vi "Configure Edge Trigger.vi"(0 "device session in":refnum<class "Device Session.lvclass">, 1 "trigger source":u8, 5 "trigger slope":T1, 7 "trigger level (V)":dbl, 9 "hysteresis (%fs)":dbl=0.25, 11 "error in":errorcluster, 12 "instance":enum16{"A", "B"}(ring)) -> (4 "device session out":refnum<class "Device Session.lvclass">, 15 "error out":errorcluster)   [LabVIEW 2021, in "Device Session.lvclass"]
doc: "Configures the edge trigger for the selected channel. You can specify the trigger level, hysteresis, and trigger slope.\n\n<B>Input Parameters</B>\n\n<B>device session in</B> is a reference to the Device Session object, which contains a session to each instrument design library used in this sample project. This parameter is obtained from the 'Open Session' VI.\n\n<B>trigger source</B> specifies the channel to monitor for trigger conditions.\n\n<B>trigger slope</B> specifies whether the oscilloscope should trigger on a rising edge or a falling edge.\n\n<B>trigger level (V)</B> specifies the voltage threshold for the trigger.\n\n<B>hysteresis (%fs)</B> specifies in volts the size of the hysteresis window on either side of the specified 'level'. The oscilloscope triggers when the 'trigger source' signal passes through the 'hysteresis level' you specify with this parameter, has the specified 'trigger slope', and passes through the specified 'level'.\n\n<B>instance</B> specifies either instance A or B of the trigger to use.\n\n<B>error in</B> describes error conditions that occur before this node runs. This input provides standard 'error in' functionality.\n\n<B>Output Parameters</B>\n\n<B>device session out</B> passes a reference to the session to the next VI.\n\n<B>error out</B> contains error information. This output provides standard 'error out' functionality."
uses:
  Device Session.lvclass
  <instrlib>/_niInstr/Data Trigger/v1/Shared/Public/Edge Configuration Trigger Slope.ctl
  Device Session.lvclass/Device Session.ctl
  <instrlib>/_niInstr/Data Trigger/v1/Shared/Public/Edge Configuration FXP(+-,18,1).ctl
  FPGA Refnum.ctl
  <vilib>/rvi/interface/nirviReadWriteControl/nirviReadWriteControl.xnode
  <vilib>/rvi/interface/Simulation/niFpgaSimulationCallBeginRW.vi
  <vilib>/rvi/errors/niLvFpgaAdjustHostInterfaceError.vi
  <instrlib>/_niInstr/Data Trigger/v1/Shared/niInstr Data Trigger v1 Shared.lvlib
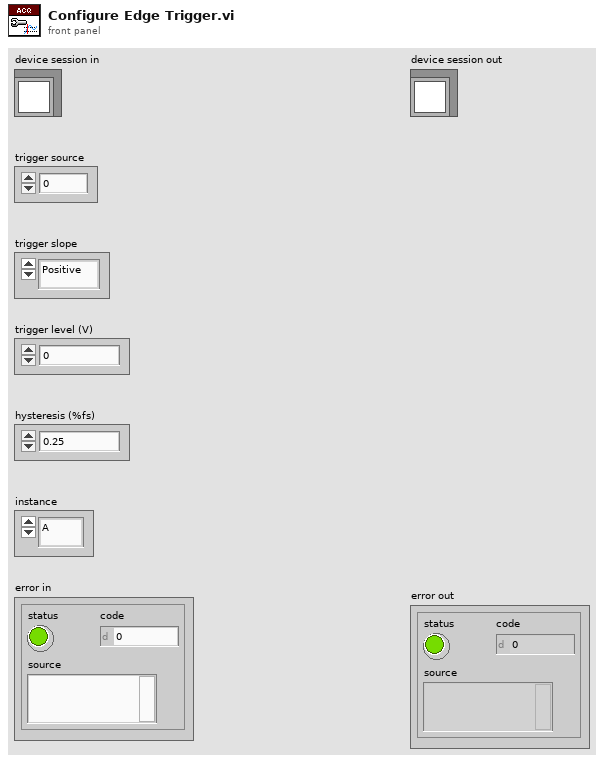
[diagram p1: front panel]
types:
  T1 = typedef "niInstr Data Trigger v1 Shared.lvlib/Edge Configuration Trigger Slope.ctl" = enum8{"Positive", "Negative"}
  T2 = typedef "niInstr Data Trigger v1 Shared.lvlib/Edge Configuration FXP(+-,18,1).ctl" = cluster{"highLevel":fxp<+/-,18,1>, "lowLevel":fxp<+/-,18,1>, "trigger slope":T1}
  T3 = typedef "Device Session.lvclass/Device Session Object.ctl" = cluster{"fpga reference":T4, "reg bus":refnum<class "niInstr FIFO Register Bus v1 Host.lvclass">, "subsystem map":refnum<class "niInstr Subsystem Map v1 Host.lvclass">, "cal data":refnum<class "niHSAI Cal Data v1 Host.lvclass">, "config":refnum<class "niHSAI Group A Config v1 Host.lvclass">, "acquisition":refnum<class "niInstr Multirecord Acquisition v1 Host.lvclass">, "number of selected acq channels":u8, "selected acq channels":bool[], "number of channels":u32, "configured channels":bool[], "acq configuration":cluster{"number of samples":u64, "number of records":u64, "pretrigger samples":u64}, "actual channel configuration":T5[], "sample clock rate (Hz)":dbl, "scaling coefficients":T9[]}
  T4 = typedef "Device Session.lvclass/FPGA Refnum.ctl" = refnum<k20>
  T5 = typedef "niHSAI Types v1 Host.lvlib/Channel Configuration.ctl" = cluster{"channel":u32, "coupling":T6, "impedance":T7, "bandwidth":T8, "vertical range":dbl, "vertical offset":dbl}
  T6 = typedef "niHSAI Types v1 Host.lvlib/Coupling.ctl" = enum8{"Default", "DC", "AC"}
  T7 = typedef "niHSAI Types v1 Host.lvlib/Impedance.ctl" = enum8{"Default", "1 mega ohm", "50 ohm"}
  T8 = typedef "niHSAI Types v1 Host.lvlib/Bandwidth.ctl" = enum8{"Default", "Full Bandwidth", "Anti-alias Filter", "150 MHz"}
  T9 = typedef "niInstr Multirecord Acquisition v1 Host.lvclass/Scaling Coefficient.ctl" = cluster{"gain":dbl, "offset":dbl}
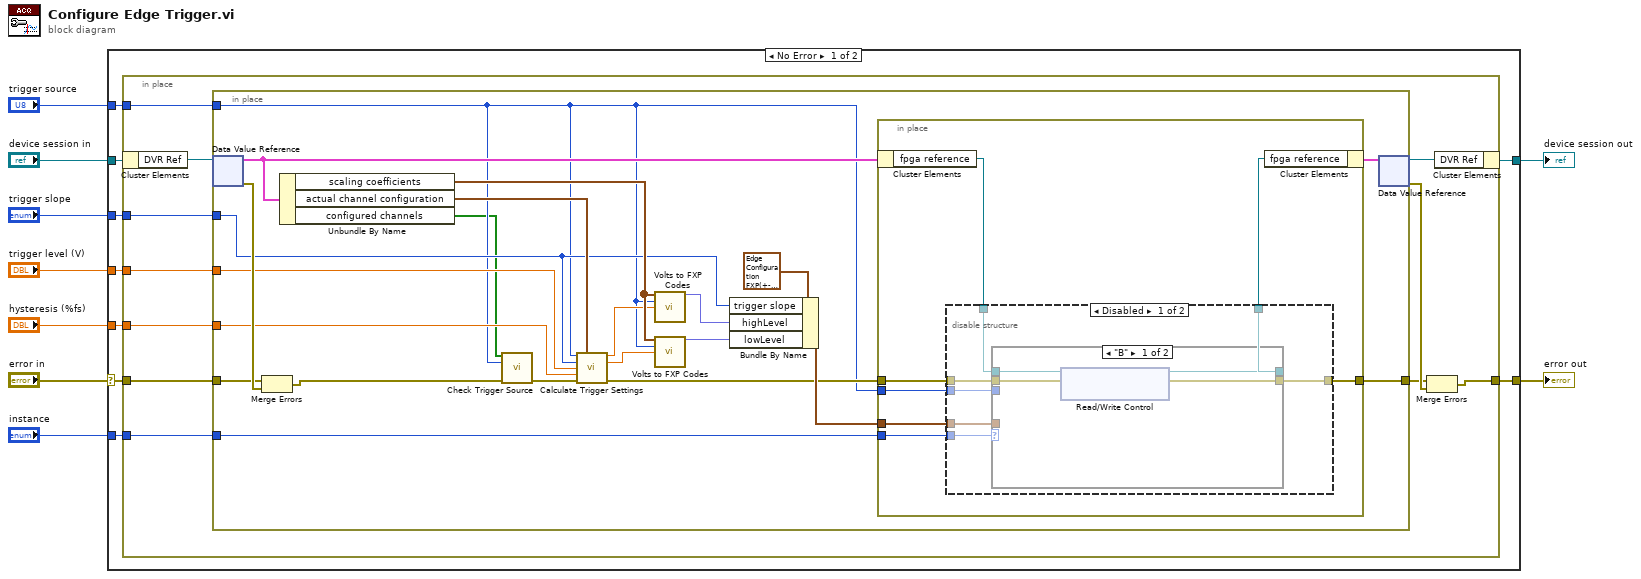
[diagram p0: block diagram]
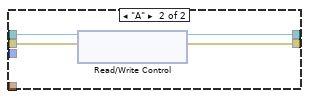
[diagram p2: hidden frame]
diagram:
  n1 = case shown="No Error" "error in" {
    selector: "error in" -> [w18 w75]
    tunnel: "device session in" -> [w11 w74]
    tunnel: [w10 w74] -> w8
    tunnel: [w12 w75] -> w9
    tunnel: "trigger source" -> [w17 _]
    tunnel: "trigger slope" -> [w16 _]
    tunnel: "trigger level (V)" -> [w15 _]
    tunnel: "hysteresis (%fs)" -> [w14 _]
    tunnel: "instance" -> [w13 _]
    frame No Error {
      n2 = in-place {
        in-place-border: w18 -> [w29]
        in-place-border: w17 -> [w28]
        in-place-border: w16 -> [w27]
        in-place-border: w15 -> [w26]
        in-place-border: w14 -> [w25]
        in-place-border: w13 -> [w23]
        in-place-border: [w21] -> w12
        n3 = in-place-cluster #1(w11) -> ("DVR Ref"=w20:refnum<data-value>)
        n4 = in-place {
          in-place-border: w29 -> [w50]
          in-place-border: w28 -> [w32]
          in-place-border: w27 -> [w34]
          in-place-border: w26 -> [w39]
          in-place-border: w25 -> [w38]
          in-place-border: w23 -> [w49]
          in-place-border: [w48] -> w22
          n5 = in-place-dvr #2(w20) -> (w36:T3, w51:errorcluster)
          n6 = Merge Errors(w50, w51) -> (w37:errorcluster)
          n7 = Unbundle By Name(w36) -> ("scaling coefficients"=w41:T9[], "actual channel configuration"=w42:T5[], "configured channels"=w30:bool[])
          n8 = call "Check Trigger Source.vi"("configured channels"=w30, "trigger source"=w32, "error in"=w37) -> ("error out"=w44:errorcluster)  [unwired: 12 in]
          n9 = call "Calculate Trigger Settings.vi"("trigger source"=w32, "actual channel configuration"=w42, "trigger slope"=w34, "level (V)"=w39, "hysteresis (%fs)"=w38, "error in"=w44) -> ("high level (V)"=w33:dbl, "low level (V)"=w40:dbl, "error out"=w43:errorcluster)  [unwired: 7 in]
          n10 = call "Volts to FXP Codes.vi"("scaling coefficients"=w41, "channel index"=w32, "level (V)"=w33) -> ("codes"=w31:fxp<+/-,18,1>)  [unwired: 12 in]
          n11 = call "Volts to FXP Codes.vi"("scaling coefficients"=w41, "channel index"=w32, "level (V)"=w40) -> ("codes"=w45:fxp<+/-,18,1>)  [unwired: 12 in]
          n12 = Bundle By Name(cluster=T2 {"highLevel"=0.0, "lowLevel"=0.0, "trigger slope"=enum."Positive"} ("configuration"), "trigger slope"=w34, "highLevel"=w31, "lowLevel"=w45) -> (w47:T2)
          n13 = in-place {
            in-place-border: w49 -> [w58]
            in-place-border: [w57] -> w48
            in-place-border: w47 -> [w56]
            in-place-border: w43 -> [w55]
            in-place-border: w32 -> [w54]
            n14 = in-place-cluster #3(w36) -> ("fpga reference"=w53:T4)
            n15 = disable-structure shown="Disabled" {
              disable-tunnel: w58 -> [w65 _]
              disable-tunnel: [w64 _] -> w57
              disable-tunnel: w56 -> [w63 _]
              disable-tunnel: w55 -> [w62 _]
              disable-tunnel: w54 -> [w61 _]
              disable-tunnel: w53 -> [w60 _]
              disable-tunnel: [w59 _] -> w52
              frame Disabled {
                n16 = case shown="\"B\"" w65 {
                  tunnel: w62 -> [w69 w73]
                  tunnel: w61 -> [_ _]
                  tunnel: [w68 w72] -> w64
                  tunnel: w63 -> [_ _]
                  tunnel: w60 -> [w67 w70]
                  tunnel: [w66 w71] -> w59
                  frame "B" {
                    n17 = xnode "Read/Write Control"("FPGA VI Reference In"=w67, "error in"=w69) -> ("FPGA VI Reference Out"=w66:T4, "error out"=w68:errorcluster)  [unwired: 1 in]
                  }
                  frame "A" {
                    n18 = xnode "Read/Write Control"("FPGA VI Reference In"=w70, "error in"=w73) -> ("FPGA VI Reference Out"=w71:T4, "error out"=w72:errorcluster)  [unwired: 1 in]
                  }
                }
              }
              frame Enabled {
              }
            }
            n19 = in-place-cluster #3("fpga reference"=w52) -> (w35:T3)
          }
          n20 = in-place-dvr #2(w35) -> (w19:refnum<data-value>, w24:errorcluster)
        }
        n21 = Merge Errors(w22, w24) -> (w21:errorcluster)
        n22 = in-place-cluster #1("DVR Ref"=w19) -> (w10:refnum<class "Device Session.lvclass">)
      }
    }
    frame Error {
    }
  }
  "error out" <- w9
  "device session out" <- w8
